vi "Retrieve Async Section group reference.vi"(8 "error in":errorcluster, 9 "Type":T3(ring), 10 "async session name":string, 11 "section item ref in":T1 format="%.0x") -> (0 "error out":errorcluster, 2 "vs group ref":T2 {"VS Refs" format="%.0x"}, 3 "section item ref out":T1 format="%.0x", 4 "Found":bool)   [LabVIEW 2019, in "HLA Custom Device System Explorer.lvlib"]
uses:
  HLA Custom Device System Explorer.lvlib
  <vilib>/NI VeriStand/Custom Device API/Custom Device Item Ref.ctl
  <vilib>/NI VeriStand/Custom Device API/Custom Device API.lvlib
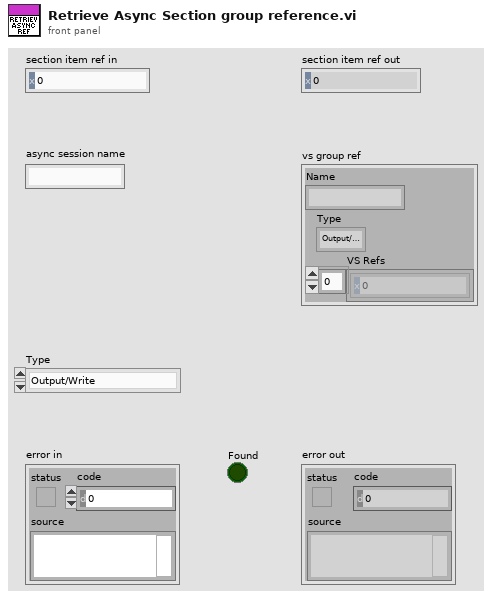
[diagram p1: front panel]
types:
  T1 = typedef "Custom Device API.lvlib/Custom Device Item Ref.ctl" = u64
  T2 = cluster{"Name":string, "Type":enum16{"Output/Write", "Input/Read", "Input/ReadWrite"}, "VS Refs":T1[]}
  T3 = enum16{"Output/Write", "Input/Read", "Input/ReadWrite"}
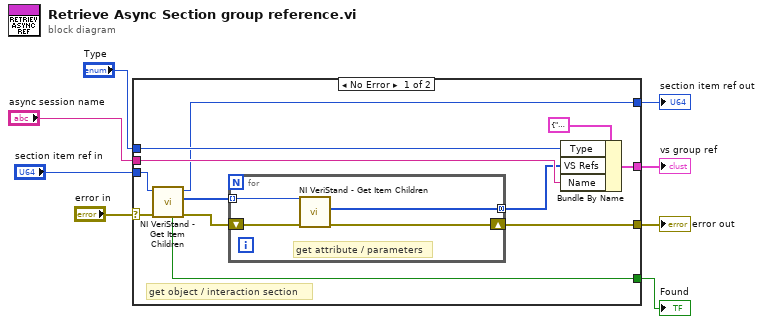
[diagram p0: block diagram]
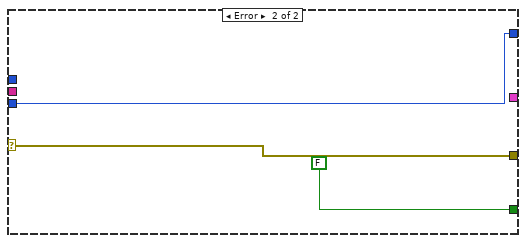
[diagram p2: hidden frame]
diagram:
  n1 = case shown="No Error" "error in" {
    selector: "error in" -> [w20 w26]
    tunnel: [w10 w26] -> w7
    tunnel: [w15 w27] -> w6
    tunnel: "section item ref in" -> [w19 w27]
    tunnel: "Type" -> [w17 _]
    tunnel: "async session name" -> [w16 _]
    tunnel: [w14 _] -> w2
    tunnel: [w13 FALSE ("Found")] -> w1
    frame No Error {
      # "get object / interaction section"
      n2 = call <vilib>:"NI VeriStand - Get Item Children.vi"("error in (no error)"=w20, "Item Ref in"=w19) -> ("error out"=w12:errorcluster, "Child Refs"=w11:T1[], "Item Ref out"=w15:T1, "Found"=w13:bool)  [unwired: 6 in]
      n3 = for {
        shift-right: [w22] -> w10
        shift-left: w12 -> [w23]
        tunnel: w11 -> [w24] mode=indexing
        tunnel: [w21] -> w9 mode=concatenating
        # "get attribute / parameters"
        n4 = call <vilib>:"NI VeriStand - Get Item Children.vi"("error in (no error)"=w23, "Item Ref in"=w24) -> ("error out"=w22:errorcluster, "Child Refs"=w21:T1[])  [unwired: 6 in, 2 out]
      }
      n5 = Bundle By Name(cluster=T2 {"Name"="", "Type"=enum."Output/Write", "VS Refs"=[]} ("Group"), "Type"=w17, "VS Refs"=w9, "Name"=w16) -> (w14:T2)
    }
    frame Error {
    }
  }
  "error out" <- w7
  "section item ref out" <- w6
  "vs group ref" <- w2
  "Found" <- w1
